vi "Handshake.vi"(8 "error in (no error)":errorcluster, 9 "timeout ms (5000)":i32=5000, 11 "WebSocket Client in":refnum<class "WebSocket Client.lvclass">) -> (0 "error out":errorcluster, 3 "WebSocket Client out":refnum<class "WebSocket Client.lvclass">)   [LabVIEW 2021, in "WebSockets.lvlib" / "WebSocket Client.lvclass"]
doc: "Performs a client-side handshake. Sends the initial handshake HTTP header and waits for response from WebSocket server. Validates received accept key from the response.\nWebSockets 2.0.1.40\nSam Sharp - MediaMongrels Ltd\nCopyright (c) 2019, MediaMongrels Ltd"
uses:
  WebSocket Client.lvclass
  D:/my_projects/projects/Algorithms/Labview/21/WebSockets/Source/WebSockets/WebSocket/WebSocket.lvclass
  WebSocket Client.lvclass/WebSocket Client.ctl
  WebSocket/WebSocket.lvclass/WebSocket.ctl
  Read URL.vi
  Sockets/Socket/Socket.lvclass
  WebSocket/WebSocket.lvclass
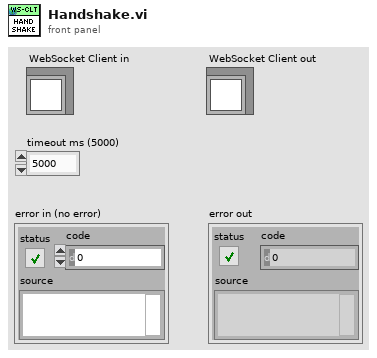
[diagram p1: front panel]
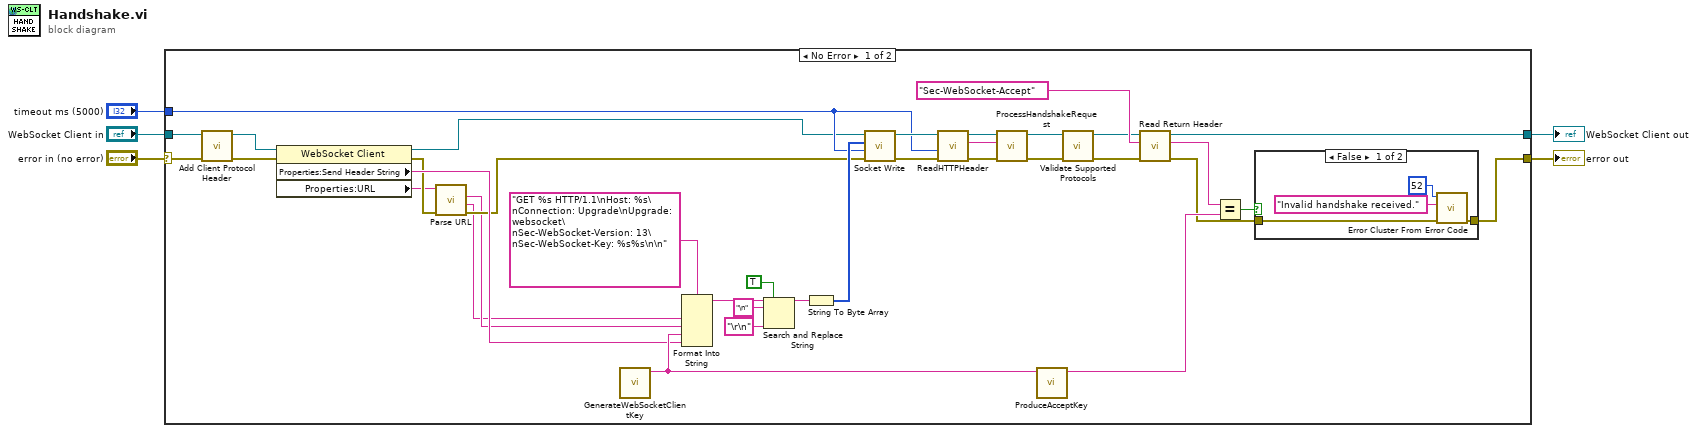
[diagram p0: block diagram]
diagram:
  n1 = case shown="No Error" "error in (no error)" {
    selector: "error in (no error)" -> [w20 w48]
    tunnel: [w21 w47] -> w5
    tunnel: "WebSocket Client in" -> [w12 w47]
    tunnel: [w28 w48] -> w2
    tunnel: "timeout ms (5000)" -> [w23 _]
    frame No Error {
      n2 = call "Add Client Protocol Header.vi"("error in (no error)"=w20, "WebSocket Client in"=w12) -> ("error out"=w13:errorcluster, "WebSocket Client out"=w11:refnum<class "WebSocket Client.lvclass">)  [unwired: 8 in]
      n3 = property class="WebSocket Client"(reference=w11, error in=w13) -> (reference out=w19:refnum<class "WebSocket Client.lvclass">, error out=w10:errorcluster, "Properties:Send Header String"=w18:string, "Properties:URL"=w9:string)
      n4 = call "Parse URL.vi"("error in (no error)"=w10, "WebSocket URL"=w9) -> ("error out"=w8:errorcluster, "URI"=w6:string, "host"=w7:string)  [unwired: 5 in, 2 out]
      n5 = call "GenerateWebSocketClientKey.vi"() -> ("WebSocket Key"=w34:string)  [unwired: 11 in]
      n6 = Format Into String(format string="GET %s HTTP/1.1\nHost: %s\nConnection: Upgrade\nUpgrade: websocket\nSec-WebSocket-Version: 13\nSec-WebSocket-Key: %s%s\n\n", w6, w7, w34, w18) -> (resulting string=w36:string)  [unwired: 2 in, 1 out]
      n7 = Search and Replace String(replace all?=TRUE ("replace all? (F)"), input string=w36, search string="\n", replace string="\r\n" ("replace string (\"\")")) -> (result string=w38:string)  [unwired: 4 in, 3 out]
      n8 = String To Byte Array(string=w38) -> (unsigned byte array=w25:u8[])
      n9 = call "Socket Write.vi"("error in (no error)"=w8, "timeout ms (5000)"=w23, "Bytes to write"=w25, "WebSocket in"=w19) -> ("error out"=w41:errorcluster, "WebSocket out"=w40:refnum<class "WebSocket Client.lvclass">)  [unwired: 4 in, 2 out]
      n10 = call "ReadHTTPHeader.vi"("error in (no error)"=w41, "timeout ms (25000)"=w23, "WebSocket in"=w40) -> ("error out"=w31:errorcluster, "HTTP Header"=w24:string, "WebSocket out"=w22:refnum<class "WebSocket Client.lvclass">)  [unwired: 6 in]
      n11 = call "ProcessHandshakeRequest.vi"("error in (no error)"=w31, "HTTP Header"=w24, "WebSocket in"=w22) -> ("error out"=w17:errorcluster, "WebSocket out"=w16:refnum<class "WebSocket Client.lvclass">)  [unwired: 4 in, 3 out]
      n12 = call "ProduceAcceptKey.vi"("Sec-WebSocket-Key"=w34) -> ("Sec-WebSocket-Accept"=w37:string)  [unwired: 10 in]
      n13 = call "Validate Supported Protocols.vi"("error in (no error)"=w17, "WebSocket In"=w16) -> ("error out"=w14:errorcluster, "WebSocket out"=w15:refnum<class "WebSocket Client.lvclass">)  [unwired: 8 in]
      n14 = call "Read Return Header.vi"("error in (no error)"=w14, "Name"="Sec-WebSocket-Accept", "WebSocket in"=w15) -> ("error out"=w29:errorcluster, "Value"=w32:string, "WebSocket out"=w21:refnum<class "WebSocket Client.lvclass">)  [unwired: 5 in, 1 out]
      n15 = Equal?(x=w32, y=w37) -> (x = y?=w30:bool)
      n16 = case shown="False" w30 {
        tunnel: w29 -> [w44 w46]
        tunnel: [w45 w46] -> w28
        frame False {
          n17 = call <vilib>:"Error Cluster From Error Code.vi"("error in (no error)"=w44, "error message (\"\")"="Invalid handshake received." ("error message (\"\")"), "error code (0)"=52) -> ("error out"=w45:errorcluster)  [unwired: 6 in]
        }
        frame True {
        }
      }
    }
    frame Error {
    }
  }
  "WebSocket Client out" <- w5
  "error out" <- w2
